vi "ClickMoveCamAdjust.vi"(0 "MoveXYBy(mm)":dbl, 1 "-X":bool, 2 "-Z":bool, 3 "+X":bool, 5 "TakePic":bool, 7 "Done":bool, 9 "MoveZBy(mm)":dbl=0.025 format="%#_13g", 11 "Error In":errorcluster, 12 "-Y":bool, 13 "+Z":bool, 14 "+Y":bool) -> (4 "Gcode":string, 6 "Image":T1(plugin-control), 15 "Error Out":errorcluster)   [LabVIEW 2019]
uses:
  <vilib>/userDefined/High Color/IMAQdx.ctl
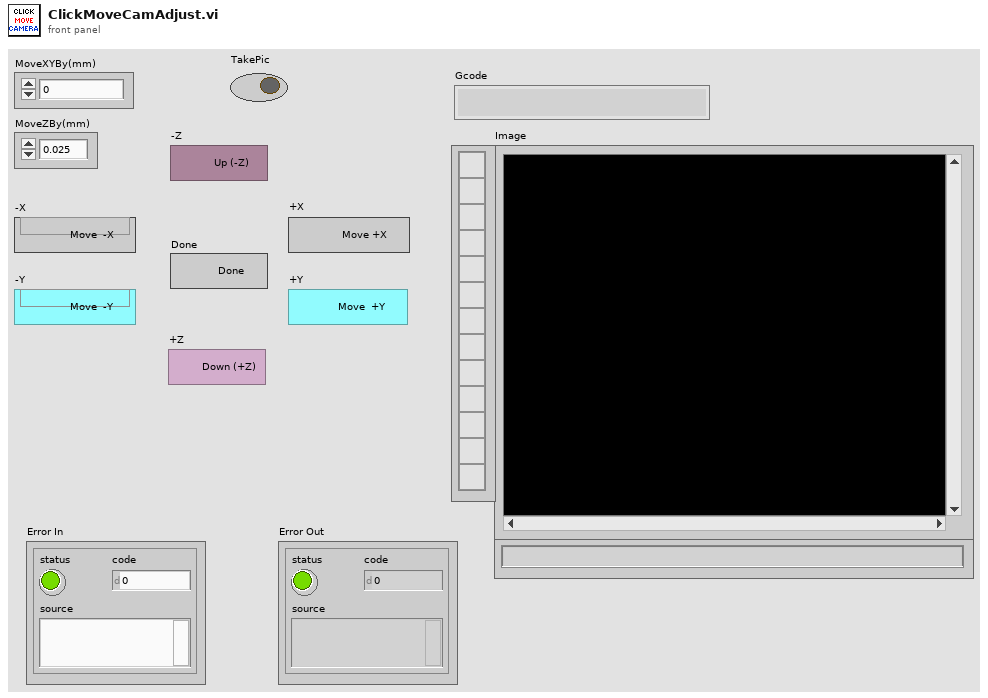
[diagram p1: front panel]
types:
  T1 = typedef "IMAQ Image.ctl" = refnum<image>
  T2 = typedef "IMAQdx.ctl" = refnum<k21>
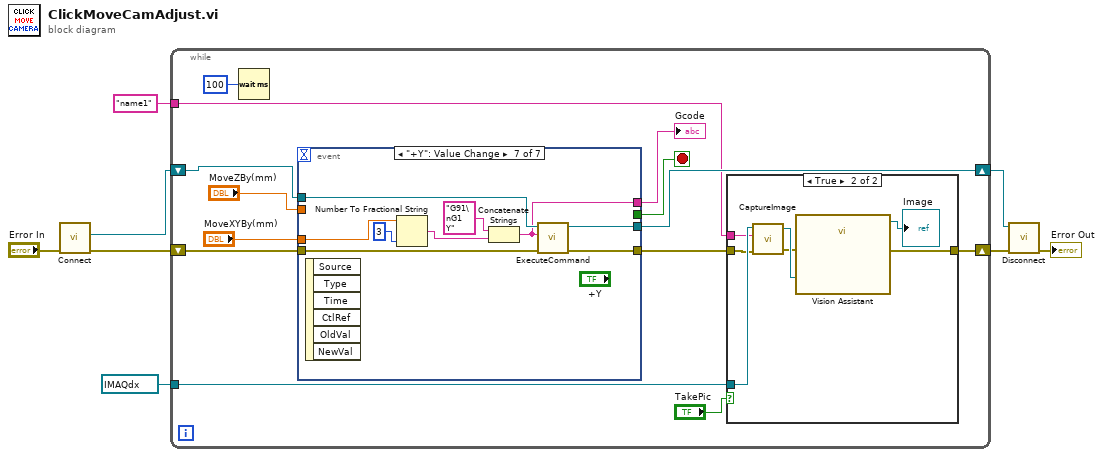
[diagram p0: block diagram]
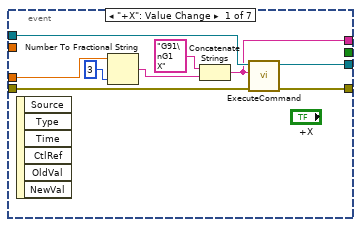
[diagram p3: hidden frame]
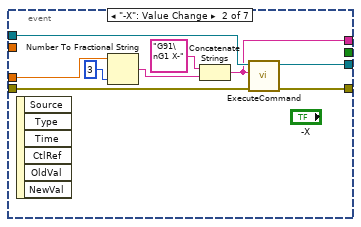
[diagram p4: hidden frame]
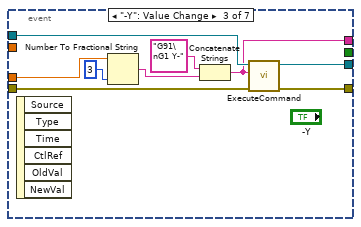
[diagram p5: hidden frame]
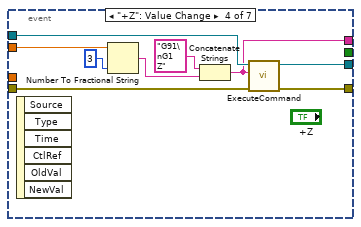
[diagram p6: hidden frame]
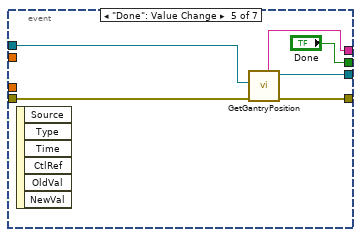
[diagram p7: hidden frame]
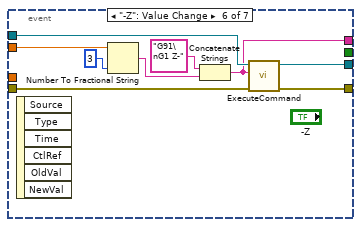
[diagram p8: hidden frame]
diagram:
  n1 = call "Connect.vi"("error in (no error)"="Error In") -> ("error out"=w5:errorcluster, "controller"=w4:refnum<k24>)  [unwired: 9 in]
  n2 = while {
    shift-right: [w11] -> w2
    shift-left: w5 -> [w21]
    shift-right: [w19] -> w1
    shift-left: w4 -> [w20]
    tunnel: "name1" ("ImageName") -> [w13]
    tunnel: T2 "cam0" ("Camera") -> [w14]
    stop <- w16 stop-if-true
    n3 = Wait (ms)(milliseconds to wait=u32 100) -> ()  [unwired: 1 out]
    n4 = event shown="[6] \"+Y\": Value Change" {
      selector: _ -> [_ _ _ _ _ _ _]
      dyn-events: _ -> [_ _ _ _ _ _ _]
      timeout: _ -> [_ _ _ _ _ _ _]
      tunnel: "MoveXYBy(mm)" -> [w35 w39 w48 _ _ _ w81]
      tunnel: w21 -> [w34 w43 w52 w61 w69 w76 w85]
      tunnel: [w33 w42 w51 w58 w66 w75 w84] -> w12
      tunnel: w20 -> [w32 w44 w53 w62 w70 w77 w86]
      tunnel: [w31 w41 w50 w59 w68 w74 w83] -> w19
      tunnel: [w30 w40 w49 w60 w67 w73 w82] -> w17
      tunnel: [_ _ _ _ "Done" _ _] -> w16
      tunnel: "MoveZBy(mm)" -> [_ _ _ w57 _ w72 _]
      event "+X": Value Change {
        n5 = event-data() -> ()  [unwired: 1 in, 6 out]
        n6 = Number To Fractional String(number=w35, precision (6)=3) -> (F-format string=w38:string)  [unwired: 2 in]
        n7 = Concatenate Strings("G91\nG1 X", w38) -> (w30:string)
        n8 = call "ExecuteCommand.vi"("error in (no error)"=w34, "Command Code"=w30, "controller in"=w32) -> ("error out"=w33:errorcluster, "controller out"=w31:refnum<k24>)  [unwired: 6 in, 1 out]
      }
      event "-X": Value Change {
        n9 = event-data() -> ()  [unwired: 1 in, 6 out]
        n10 = Number To Fractional String(number=w39, precision (6)=3) -> (F-format string=w47:string)  [unwired: 2 in]
        n11 = Concatenate Strings("G91\nG1 X-", w47) -> (w40:string)
        n12 = call "ExecuteCommand.vi"("error in (no error)"=w43, "Command Code"=w40, "controller in"=w44) -> ("error out"=w42:errorcluster, "controller out"=w41:refnum<k24>)  [unwired: 6 in, 1 out]
      }
      event "-Y": Value Change {
        n13 = event-data() -> ()  [unwired: 1 in, 6 out]
        n14 = Number To Fractional String(number=w48, precision (6)=3) -> (F-format string=w56:string)  [unwired: 2 in]
        n15 = Concatenate Strings("G91\nG1 Y-", w56) -> (w49:string)
        n16 = call "ExecuteCommand.vi"("error in (no error)"=w52, "Command Code"=w49, "controller in"=w53) -> ("error out"=w51:errorcluster, "controller out"=w50:refnum<k24>)  [unwired: 6 in, 1 out]
      }
      event "+Z": Value Change {
        n17 = event-data() -> ()  [unwired: 1 in, 6 out]
        n18 = Number To Fractional String(number=w57, precision (6)=3) -> (F-format string=w65:string)  [unwired: 2 in]
        n19 = Concatenate Strings("G91\nG1 Z", w65) -> (w60:string)
        n20 = call "ExecuteCommand.vi"("error in (no error)"=w61, "Command Code"=w60, "controller in"=w62) -> ("error out"=w58:errorcluster, "controller out"=w59:refnum<k24>)  [unwired: 6 in, 1 out]
      }
      event "Done": Value Change {
        n21 = event-data() -> ()  [unwired: 1 in, 6 out]
        n22 = call "GetGantryPosition.vi"("error in (no error)"=w69, "Controller In"=w70) -> ("error out"=w66:errorcluster, "controller out"=w68:refnum<k24>, "Position_XYZ"=w67:string)  [unwired: 3 in, 4 out]
      }
      event "-Z": Value Change {
        n23 = event-data() -> ()  [unwired: 1 in, 6 out]
        n24 = Number To Fractional String(number=w72, precision (6)=3) -> (F-format string=w80:string)  [unwired: 2 in]
        n25 = Concatenate Strings("G91\nG1 Z-", w80) -> (w73:string)
        n26 = call "ExecuteCommand.vi"("error in (no error)"=w76, "Command Code"=w73, "controller in"=w77) -> ("error out"=w75:errorcluster, "controller out"=w74:refnum<k24>)  [unwired: 6 in, 1 out]
      }
      event "+Y": Value Change {
        n27 = event-data() -> ()  [unwired: 1 in, 6 out]
        n28 = Number To Fractional String(number=w81, precision (6)=3) -> (F-format string=w89:string)  [unwired: 2 in]
        n29 = Concatenate Strings("G91\nG1 Y", w89) -> (w82:string)
        n30 = call "ExecuteCommand.vi"("error in (no error)"=w85, "Command Code"=w82, "controller in"=w86) -> ("error out"=w84:errorcluster, "controller out"=w83:refnum<k24>)  [unwired: 6 in, 1 out]
      }
    }
    "Gcode" <- w17
    n31 = case shown="True" "TakePic" {
      tunnel: w14 -> [_ w29]
      tunnel: w13 -> [_ w28]
      tunnel: w12 -> [w22 w27]
      tunnel: [w22 w24] -> w11
      frame False {
      }
      frame True {
        n32 = call "CaptureImage.vi"("Camera"=w29, "ImageName"=w28, "error in (no error)"=w27) -> ("Image"=w26:T1, "error out"=w25:errorcluster)  [unwired: 4 in]
        n33 = call "Vision Assistant"("Image In"=w26, "error in"=w25) -> ("Image Out"=→"Image":T1, "error out"=w24:errorcluster)  [unwired: 24 in]
      }
    }
  }
  n34 = call "Disconnect.vi"("error in (no error)"=w2, "controller"=w1) -> ("error out"=→"Error Out":errorcluster)  [unwired: 9 in]
